vi "Data Logging Write to Measurement File DAQ.vi"() -> ()   [LabVIEW 2020]
uses:
  <vilib>/DAQmx/read.llb/DAQmx Read (Analog Wfm 1Chan NSamp).vi
  <vilib>/DAQmx/create/channels.llb/DAQmx Create Channel (AI-Voltage-Basic).vi
  <vilib>/DAQmx/configure/timing.llb/DAQmx Timing (Sample Clock).vi
  <vilib>/DAQmx/miscellaneous.llb/DAQmx Fill In Error Info.vi
panel:
  out "Waveform Graph":waveform(dbl)(graph)
  in  "rate":dbl=1000.0 format="%0.2f"
  in  "samples per channel":i32=1000
  in  "sample mode":i32(ring)=10178 items=["Finite Samples"=10178, "Continuous Samples"=10123, "Hardware Timed Single Point"=12522]
  in  "physical channels":tag
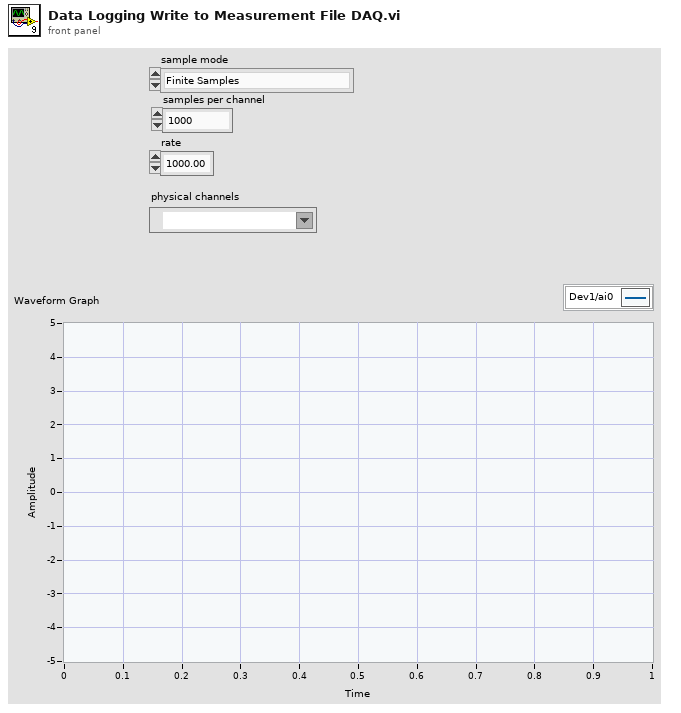
[diagram p1: front panel]
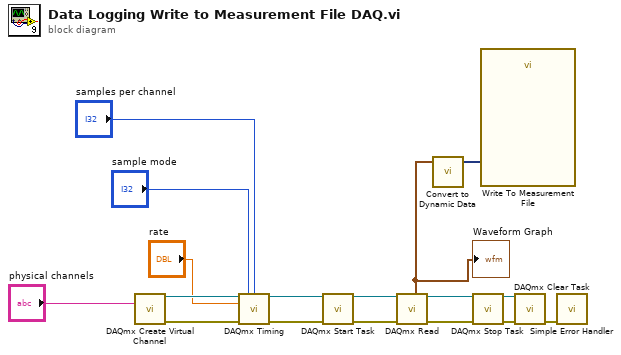
[diagram p0: block diagram]
diagram:
  n1 = call-poly <vilib>:"DAQmx Create Virtual Channel.vi"("physical channels"="physical channels") -> ("task out"=w9:refnum<k21>, "error out"=w8:errorcluster)  [unwired: 13 in]
  n2 = call-poly <vilib>:"DAQmx Timing.vi"("task/channels in"=w9, "sample mode"="sample mode", "samples per channel"="samples per channel", "rate"="rate", "error in"=w8) -> ("task out"=w4:refnum<k21>, "error out"=w3:errorcluster)  [unwired: 9 in]
  n3 = call <vilib>:"DAQmx Start Task.vi"("task/channels in"=w4, "error in"=w3) -> ("task out"=w16:refnum<k21>, "error out"=w15:errorcluster)  [unwired: 12 in]
  n4 = call-poly <vilib>:"DAQmx Read.vi"("task/channels in"=w16, "error in"=w15) -> ("task out"=w14:refnum<k21>, "data"=w2:waveform(dbl), "error out"=w13:errorcluster)  [unwired: 11 in]
  "Waveform Graph" <- w2
  n5 = call "Convert to Dynamic Data"("Waveform"=w2) -> ("Dynamic Data Type"=w1:dynamicdata)  [unwired: 3 in]
  n6 = call <vilib>:"DAQmx Stop Task.vi"("task/channels in"=w14, "error in"=w13) -> ("task out"=w12:refnum<k21>, "error out"=w11:errorcluster)  [unwired: 12 in]
  n7 = call "Write To Measurement File"("Signals"=w1) -> ()  [unwired: 16 in, 3 out]
  n8 = call <vilib>:"DAQmx Clear Task.vi"("task in"=w12, "error in"=w11) -> ("error out"=w10:errorcluster)  [unwired: 13 in]
  n9 = call <vilib>:"Simple Error Handler.vi"("error in (no error)"=w10) -> ()  [unwired: 4 in, 5 out]
